vi "Enquene Function.vi"(8 "error in (no error)":errorcluster, 10 "Queue":refnum<queue>) -> (0 "error out":errorcluster, 2 "Data":variant, 3 "Message":string)   [LabVIEW 2020]
uses:
  Def/Queue_Def.ctl
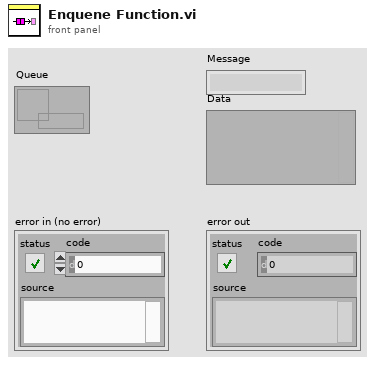
[diagram p1: front panel]
types:
  T1 = typedef "Queue_Def.ctl" = cluster{"Message":string, "Data":variant}
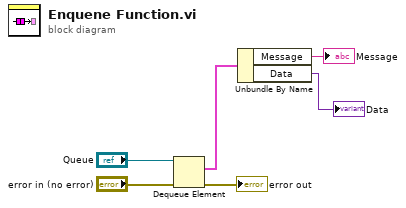
[diagram p0: block diagram]
diagram:
  n1 = Dequeue Element(queue="Queue", error in (no error)="error in (no error)") -> (element=w1:T1, error out=→"error out":errorcluster)  [unwired: 1 in, 2 out]
  n2 = Unbundle By Name(w1) -> ("Message"=→"Message":string, "Data"=→"Data":variant)
